vi "Configure Dual Channel Impulse Response.vi"(0 "VISA resource name":refnum<visa-resource-name>, 1 "Impulse Response Stop Time (0 s)":dbl, 2 "Impulse Response Stop Window (0: irwNone)":i32(ring) items=["irwNone", "irw5pct", "irw10pct", "irw20pct", "irw30pct"], 5 "Analyzer (0: A0)":i32(ring) items=["A0", "A1"], 7 "Enable Calculate Impulse Response (T: Enable)":bool=TRUE, 9 "Impulse Response Start Time (0 s)":dbl, 11 "error in (no error)":errorcluster, 12 "Impulse Response Start Window (0: irwNone)":i32(ring) items=["irwNone", "irw5pct", "irw10pct", "irw20pct", "irw30pct"]) -> (4 "VISA resource name out":refnum<visa-resource-name>, 15 "error out":errorcluster)   [LabVIEW 2014, in "Stanford Research SR1.lvlib"]
doc: "Configures the attributes for the Dual Channel Impulse Response."
uses:
  Stanford Research SR1.lvlib
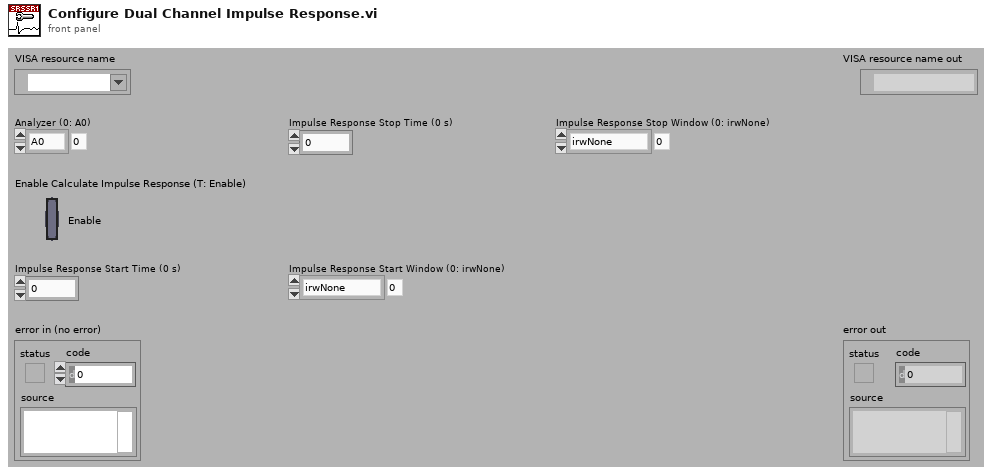
[diagram p1: front panel]
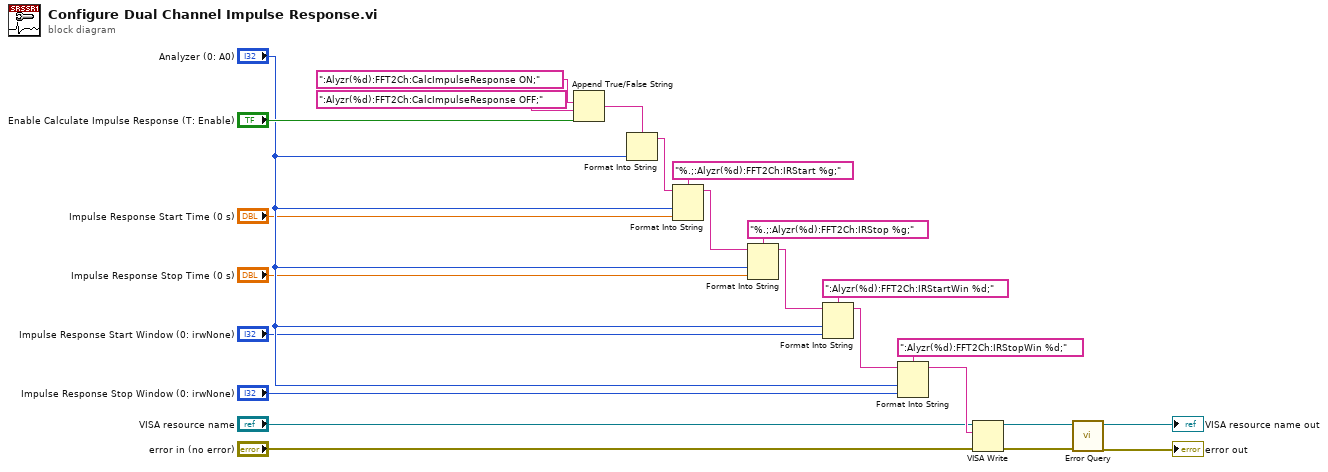
[diagram p0: block diagram]
diagram:
  n1 = Append True/False String(1:"Enable Calculate Impulse Response (T: Enable)", 2:":Alyzr(%d):FFT2Ch:CalcImpulseResponse OFF;", 3:":Alyzr(%d):FFT2Ch:CalcImpulseResponse ON;") -> (0:w7:string)  [unwired: 1 in]
  n2 = Format Into String(format string=w7, "Analyzer (0: A0)") -> (resulting string=w5:string)  [unwired: 2 in, 1 out]
  n3 = Format Into String(format string="%.;:Alyzr(%d):FFT2Ch:IRStart %g;", initial string=w5, "Analyzer (0: A0)", "Impulse Response Start Time (0 s)") -> (resulting string=w20:string)  [unwired: 1 in, 1 out]
  n4 = Format Into String(format string="%.;:Alyzr(%d):FFT2Ch:IRStop %g;", initial string=w20, "Analyzer (0: A0)", "Impulse Response Stop Time (0 s)") -> (resulting string=w18:string)  [unwired: 1 in, 1 out]
  n5 = Format Into String(format string=":Alyzr(%d):FFT2Ch:IRStartWin %d;", initial string=w18, "Analyzer (0: A0)", "Impulse Response Start Window (0: irwNone)") -> (resulting string=w16:string)  [unwired: 1 in, 1 out]
  n6 = Format Into String(format string=":Alyzr(%d):FFT2Ch:IRStopWin %d;", initial string=w16, "Analyzer (0: A0)", "Impulse Response Stop Window (0: irwNone)") -> (resulting string=w14:string)  [unwired: 1 in, 1 out]
  n7 = VISA Write(VISA resource name="VISA resource name", write buffer=w14, error in (no error)="error in (no error)") -> (VISA resource name out=w11:refnum<visa-resource-name>, error out=w10:errorcluster)  [unwired: 1 out]
  n8 = call "Error Query.vi"("error in (no error)"=w10, "VISA resource name"=w11) -> ("error out"=→"error out":errorcluster, "VISA resource name out"=→"VISA resource name out":refnum<visa-resource-name>)  [unwired: 6 in, 2 out]
